vi "setValue.vi"(8 "error in (no error)":errorcluster, 10 "Value in":refnum<class "IBaseObject.lvclass">, 11 "IProperty in":refnum<class "IProperty.lvclass">) -> (0 "error out":errorcluster, 3 "IProperty out":refnum<class "IProperty.lvclass">)   [LabVIEW 2022 SP3, in "openDAQ.lvlib" / "IBaseObject.lvlib" / "IProperty.lvlib" / "IProperty.lvclass"]
uses:
  <instrlib>/openDAQ/Public/Classes/IProperty/IProperty.lvclass
  C:/Program Files (x86)/National Instruments/LabVIEW 2022/instr.lib/openDAQ/Public/Classes/IBaseObject/IBaseObject.lvclass
  <instrlib>/openDAQ/Public/Classes/IBaseObject/IBaseObject.lvclass
  <instrlib>/openDAQ/Public/Classes/IBaseObject/IBaseObject.lvclass/IBaseObject.ctl
  <instrlib>/openDAQ/Public/Classes/IBaseObject/Accessor/Read reference.vi
  <instrlib>/openDAQ/Public/Classes/IProperty/IProperty.lvclass/IProperty.ctl
  <instrlib>/openDAQ/Binaries/Windows/x86/copendaq32.dll
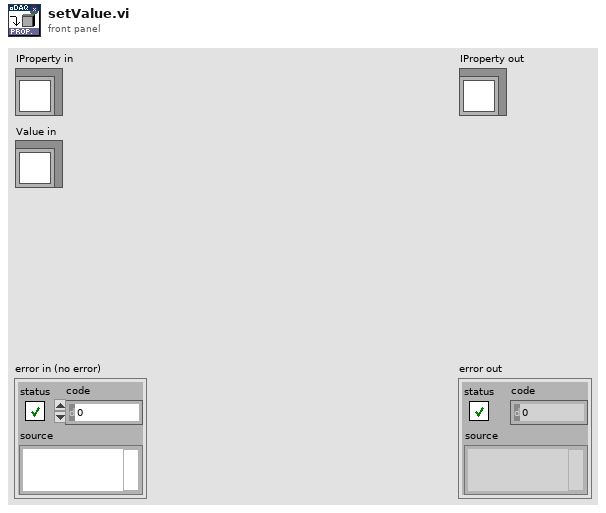
[diagram p1: front panel]
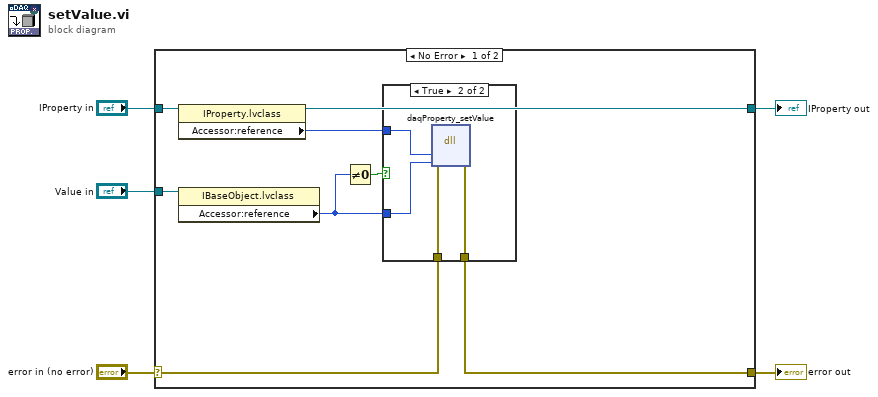
[diagram p0: block diagram]
diagram:
  n1 = case shown="No Error" "error in (no error)" {
    selector: "error in (no error)" -> [w12 w20]
    tunnel: [w11 w20] -> w4
    tunnel: [w8 w19] -> w2
    tunnel: "IProperty in" -> [w13 w19]
    tunnel: "Value in" -> [w10 _]
    frame No Error {
      n2 = property class="IProperty.lvclass"(reference=w13) -> (reference out=w8:refnum<class "IProperty.lvclass">, "Accessor:reference"=w9:i64)  [unwired: 1 in, 1 out]
      n3 = property class="IBaseObject.lvclass"(reference=w10) -> ("Accessor:reference"=w7:i64)  [unwired: 1 in, 2 out]
      n4 = Not Equal To 0?(x=w7) -> (x != 0?=w6:bool)
      n5 = case shown="True" w6 {
        tunnel: w12 -> [w14 w18]
        tunnel: [w14 w17] -> w11
        tunnel: w9 -> [_ w16]
        tunnel: w7 -> [_ w15]
        frame False {
        }
        frame True {
          n6 = dll-call lib="C:/Program Files (x86)/National Instruments/LabVIEW 2022/instr.lib/openDAQ/Binaries/Windows/x86/copendaq*.*" fn="daqProperty_setValue"(error in=w18, "property"=w16, "value"=w15) -> (error out=w17:errorcluster)  [unwired: 5 in, 1 out]
        }
      }
    }
    frame Error {
    }
  }
  "error out" <- w4
  "IProperty out" <- w2
